vi "Initialization VI.vi"(8 "error in (no error)":errorcluster, 10 "Custom XML":string, 11 "Device Item Ref in":T1 format="%.0x") -> (0 "error out":errorcluster, 3 "Device Item Ref out":T1 format="%.0x")   [LabVIEW 2015, in "Protection and Counter Addon System Explorer.lvlib"]
uses:
  Protection and Counter Addon System Explorer.lvlib
  <vilib>/NI Veristand/Custom Device API/Custom Device Item Ref.ctl
  <vilib>/NI Veristand/Custom Device API/Custom Device Channel.ctl
  <vilib>/NI Veristand/Custom Device API/Custom Device Channel Type.ctl
  Shared/SubVIs/GUID Lookup.vi
  <vilib>/NI VeriStand/Custom Device API/Custom Device API.lvlib
  Shared/Protection and Counter Addon Shared.lvlib
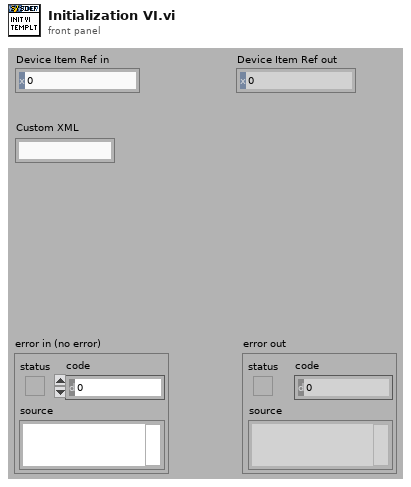
[diagram p1: front panel]
types:
  T1 = typedef "Custom Device API.lvlib/Custom Device Item Ref.ctl" = u64
  T2 = typedef "Custom Device API.lvlib/Custom Device Channel.ctl" = cluster{"Type":T3, "Units":string, "Default Value":dbl, "Faultable":bool, "Scalable":bool}
  T3 = typedef "Custom Device API.lvlib/Custom Device Channel Type.ctl" = enum16{"Input", "Output"}
  T4 = typedef "Protection and Counter Addon Shared.lvlib/XNET Settings.ctl" = cluster{"Database":refnum<k21>, "Cluster":refnum<k21>, "Port":string, "Baud rate [Bd]":u64, "Termination":u32, "CAN I/O Mode":u32, "FD Baud rate [Bd]":u64, "Priority":i32, "Use Legacy":bool}
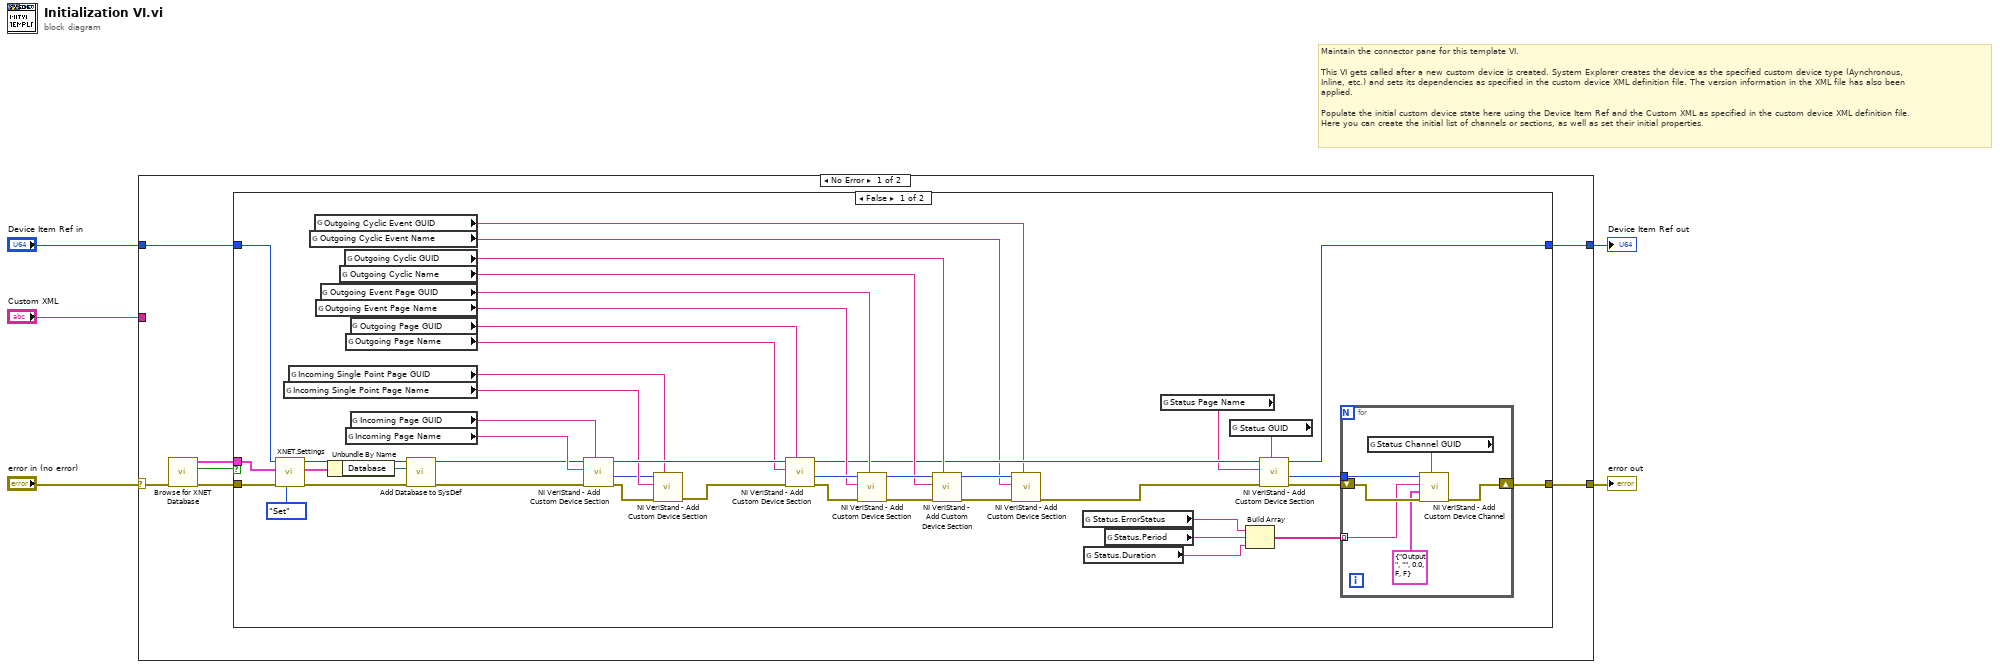
[diagram p0: block diagram]
diagram:
  # "Maintain the connector pane for this template VI.\n\nThis VI gets called after a new custom device is created. System Explorer creates the device as the specified custom device type (Aynchronous, Inline, etc.) and sets its dependencies as specified in the custom device XML definition file. The version information in the XML file has also been applied.\n\nPopulate the initial custom device state here using the Device Item Ref and the Custom XML as specified in the custom device XML definition file. Here you can create the initial list of channels or sections, as well as set their initial properties."
  n1 = case shown="No Error" "error in (no error)" {
    selector: "error in (no error)" -> [w10 w66]
    tunnel: [w12 w66] -> w5
    tunnel: [w11 w65] -> w3
    tunnel: "Device Item Ref in" -> [w8 w65]
    tunnel: "Custom XML" -> [_ _]
    frame No Error {
      n2 = call "Browse for XNET Database.vi"("error in (no error)"=w10) -> ("error out"=w9:errorcluster, "Cancel Out"=w7:bool, "XNET Settings"=w6:T4)  [unwired: 8 in]
      n3 = case shown="False" w7 {
        tunnel: [w26 w64] -> w12
        tunnel: [w27 w63] -> w11
        tunnel: w9 -> [w49 w64]
        tunnel: w8 -> [w47 w63]
        tunnel: w6 -> [w45 _]
        frame False {
          n4 = call "XNET.Settings.vi"("Action"=enum8{"Get", "Set"}."Set", "error in (no error)"=w49, "XNET Settings"=w45, "Parent Ref in"=w47) -> ("error out"=w48:errorcluster, "XNET Settings"=w44:T4, "Item Ref out"=w46:T1)  [unwired: 5 in]
          n5 = global read "GUID Lookup.vi" "Incoming Single Point Page Name"() -> (w31:string)
          n6 = global read "GUID Lookup.vi" "Incoming Single Point Page GUID"() -> (w32:string)
          n7 = global read "GUID Lookup.vi" "Outgoing Cyclic Event Name"() -> (w15:string)
          n8 = global read "GUID Lookup.vi" "Outgoing Cyclic Event GUID"() -> (w16:string)
          n9 = global read "GUID Lookup.vi" "Outgoing Event Page Name"() -> (w36:string)
          n10 = global read "GUID Lookup.vi" "Outgoing Event Page GUID"() -> (w37:string)
          n11 = Unbundle By Name(w44) -> ("Database"=w43:refnum<k21>)
          n12 = global read "GUID Lookup.vi" "Outgoing Cyclic Name"() -> (w34:string)
          n13 = global read "GUID Lookup.vi" "Outgoing Cyclic GUID"() -> (w35:string)
          n14 = global read "GUID Lookup.vi" "Outgoing Page Name"() -> (w53:string)
          n15 = global read "GUID Lookup.vi" "Incoming Page Name"() -> (w52:string)
          n16 = global read "GUID Lookup.vi" "Outgoing Page GUID"() -> (w54:string)
          n17 = global read "GUID Lookup.vi" "Incoming Page GUID"() -> (w56:string)
          n18 = call "Add Database to SysDef.vi"("error in"=w48, "DB Alias"=w43, "Item Ref in"=w46) -> ("error out"=w51:errorcluster, "Item Ref out"=w50:T1)  [unwired: 7 in]
          n19 = call <vilib>:"NI VeriStand - Add Custom Device Section.vi"("GUID (Default Section)"=w56, "error in (no error)"=w51, "Section Name"=w52, "Parent Ref in"=w50) -> ("error out"=w13:errorcluster, "Section Ptr"=w14:T1, "Parent Ref out"=w55:T1)  [unwired: 4 in, 1 out]
          n20 = call <vilib>:"NI VeriStand - Add Custom Device Section.vi"("GUID (Default Section)"=w32, "error in (no error)"=w13, "Section Name"=w31, "Parent Ref in"=w14) -> ("error out"=w33:errorcluster)  [unwired: 4 in, 3 out]
          n21 = call <vilib>:"NI VeriStand - Add Custom Device Section.vi"("GUID (Default Section)"=w54, "error in (no error)"=w33, "Section Name"=w53, "Parent Ref in"=w55) -> ("error out"=w39:errorcluster, "Section Ptr"=w41:T1, "Parent Ref out"=w28:T1)  [unwired: 4 in, 1 out]
          n22 = call <vilib>:"NI VeriStand - Add Custom Device Section.vi"("GUID (Default Section)"=w37, "error in (no error)"=w39, "Section Name"=w36, "Parent Ref in"=w41) -> ("error out"=w40:errorcluster, "Parent Ref out"=w38:T1)  [unwired: 4 in, 2 out]
          n23 = call <vilib>:"NI VeriStand - Add Custom Device Section.vi"("GUID (Default Section)"=w35, "error in (no error)"=w40, "Section Name"=w34, "Parent Ref in"=w38) -> ("error out"=w18:errorcluster, "Parent Ref out"=w19:T1)  [unwired: 4 in, 2 out]
          n24 = call <vilib>:"NI VeriStand - Add Custom Device Section.vi"("GUID (Default Section)"=w16, "error in (no error)"=w18, "Section Name"=w15, "Parent Ref in"=w19) -> ("error out"=w17:errorcluster)  [unwired: 4 in, 3 out]
          n25 = global read "GUID Lookup.vi" "Status.ErrorStatus"() -> (w25:string)
          n26 = global read "GUID Lookup.vi" "Status.Duration"() -> (w23:string)
          n27 = global read "GUID Lookup.vi" "Status.Period"() -> (w24:string)
          n28 = global read "GUID Lookup.vi" "Status Page Name"() -> (w20:string)
          n29 = global read "GUID Lookup.vi" "Status GUID"() -> (w21:string)
          n30 = Build Array(w25, w24, w23) -> (w22:string[])
          n31 = call <vilib>:"NI VeriStand - Add Custom Device Section.vi"("GUID (Default Section)"=w21, "error in (no error)"=w17, "Section Name"=w20, "Parent Ref in"=w28) -> ("error out"=w29:errorcluster, "Section Ptr"=w30:T1, "Parent Ref out"=w27:T1)  [unwired: 4 in, 1 out]
          n32 = for {
            tunnel: w30 -> [w62]
            shift-right: [w60] -> w26
            shift-left: w29 -> [w61]
            tunnel: w22 -> [w57] mode=indexing
            n33 = global read "GUID Lookup.vi" "Status Channel GUID"() -> (w59:string)
            n34 = call <vilib>:"NI VeriStand - Add Custom Device Channel.vi"("GUID (Default Channel)"=w59, "error in (no error)"=w61, "Channel"=T2 {"Type"=enum."Output", "Units"="", "Default Value"=0.0, "Faultable"=FALSE, "Scalable"=FALSE}, "Channel Name"=w57, "Parent Ref in"=w62) -> ("error out"=w60:errorcluster)  [unwired: 3 in, 3 out]
          }
        }
        frame True {
        }
      }
    }
    frame Error {
    }
  }
  "error out" <- w5
  "Device Item Ref out" <- w3
